vi "Get Prescale Factor.vi"(8 "error in (no error)":errorcluster, 10 "Prescaler (Trigger input)":i32(ring) items=["Trigger input", "Output AB", "Output CD", "Output EF", "Output GH"], 11 "VISA resource name":refnum<visa-resource-name>) -> (0 "error out":errorcluster, 2 "Prescale Factor":i32, 3 "VISA resource name out":refnum<visa-resource-name>, 4 "Device Errors":cluster{"code":i32, "Text":string}[](array[cluster]))   [LabVIEW 2014, in "Stanford Research DG645 - Driver.lvlib"]
doc: "Trigger Command: PRES? i\nInstrument Error Check\n\nQuery the prescale factor for channel i. The parameter i selects the prescaler according to the following table:\n\ni Prescaler\n0 Trigger input \n1 Output AB\n2 Output CD\n3 Output EF\n4 Output GH\n\nIf prescaling is enabled and i equals 0 (Trigger input), every j'th trigger will initiate a delay cycle. If prescaling is enabled and i equals 1...4 (Output), the output will be enabled only every j'th delay cycle."
uses:
  Stanford Research DG645 - Driver.lvlib
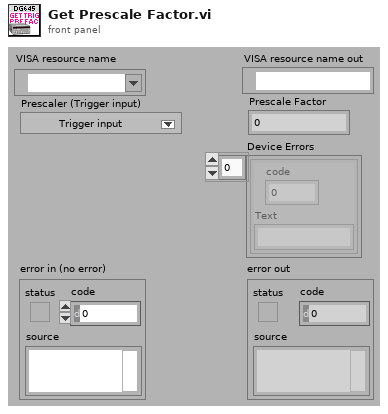
[diagram p1: front panel]
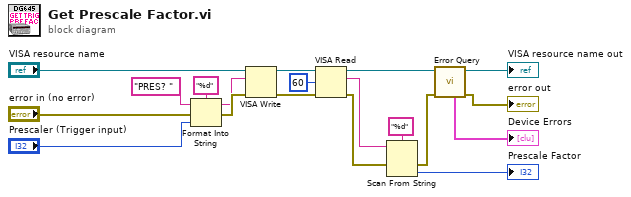
[diagram p0: block diagram]
diagram:
  n1 = Format Into String(format string="%d", initial string="PRES? " ("command"), error in="error in (no error)", "Prescaler (Trigger input)") -> (resulting string=w15:string, error out=w16:errorcluster)
  n2 = VISA Write(VISA resource name="VISA resource name", write buffer=w15, error in (no error)=w16) -> (VISA resource name out=w12:refnum<visa-resource-name>, error out=w11:errorcluster)  [unwired: 1 out]
  n3 = VISA Read(VISA resource name=w12, byte count=u32 60, error in (no error)=w11) -> (VISA resource name out=w10:refnum<visa-resource-name>, read buffer=w7:string, error out=w3:errorcluster)  [unwired: 1 out]
  n4 = Scan From String(format string="%d", input string=w7, error in=w3) -> (error out=w2:errorcluster, output 1=→"Prescale Factor":i32)  [unwired: 2 in, 2 out]
  n5 = call "Error Query.vi"("error in (no error)"=w2, "VISA resource name"=w10) -> ("error out"=→"error out":errorcluster, "VISA resource name out"=→"VISA resource name out":refnum<visa-resource-name>, "Device Errors"=→"Device Errors":cluster{"code":i32, "Text":string}[])  [unwired: 7 in]
